vi "PXI-Compute DI Skip Samples.vi"(0 "AO Tasks":T1[](array[typedef]), 7 "DI Tasks":T1[](array[typedef]), 11 "error in (no error)":errorcluster) -> (4 "Skip Samples":i32, 15 "error out":errorcluster)   [LabVIEW 2020]
doc: "Determines the number of AI samples to skip in order to register AO and AI (accounting for the latencies of the 24-bit boards)."
uses:
  Type Defs/Task Struct.ctl
  PXI Globals.vi
panel:
  out "Any 16-bit AI?":bool
  out "Any 16-bit AO?":bool
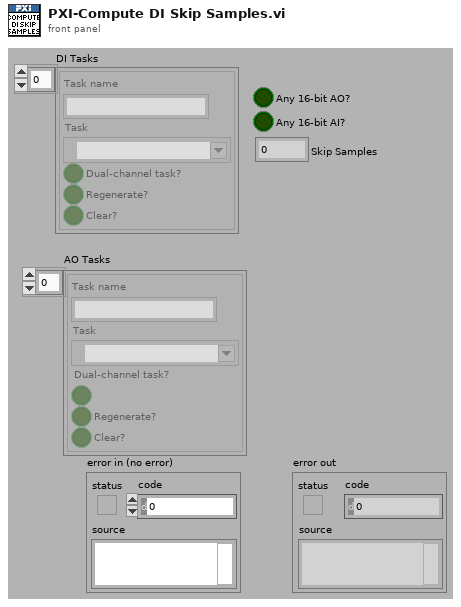
[diagram p1: front panel]
types:
  T1 = typedef "Task Struct.ctl" = cluster{"Task name":string, "Task":refnum<k21>, "Dual-channel task?":bool, "Regenerate?":bool, "Clear?":bool}
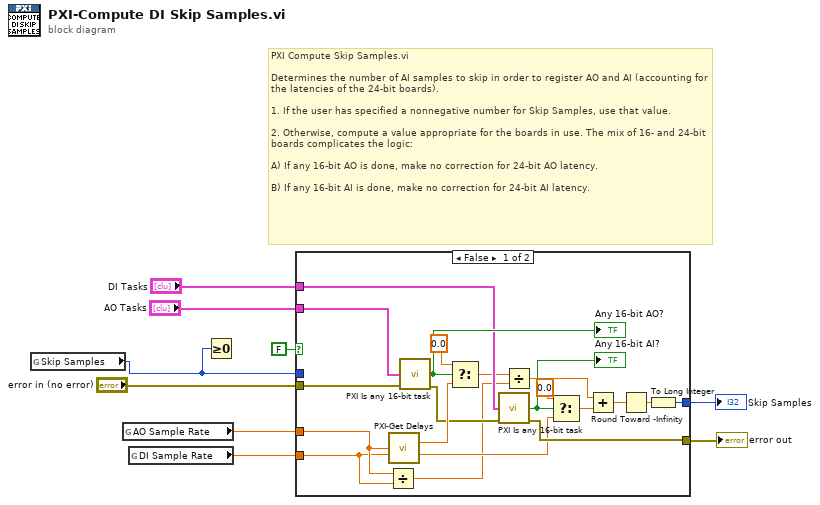
[diagram p0: block diagram]
diagram:
  # "PXI Compute Skip Samples.vi\n\nDetermines the number of AI samples to skip in order to register AO and AI (accounting for the latencies of the 24-bit boards). \n\n1. If the user has specified a nonnegative number for Skip Samples, use that value. \n\n2. Otherwise, compute a value appropriate for the boards in use. The mix of 16- and 24-bit boards complicates the logic:\n\nA) If any 16-bit AO is done, make no correction for 24-bit AO latency.\n\nB) If any 16-bit AI is done, make no correction for 24-bit AI latency."
  n1 = global read "PXI Globals.vi" "Skip Samples"() -> (w7:i32)
  n2 = global read "PXI Globals.vi" "AO Sample Rate"() -> (w5:dbl)
  n3 = global read "PXI Globals.vi" "DI Sample Rate"() -> (w4:dbl)
  n4 = Greater Or Equal To 0?(x=w7) -> ()  [unwired: 1 out]
  n5 = case shown="False" FALSE {
    tunnel: "error in (no error)" -> [w10 w31]
    tunnel: [w27 w30] -> w3
    tunnel: [w20 w31] -> w9
    tunnel: w7 -> [_ w30]
    tunnel: "AO Tasks" -> [w26 _]
    tunnel: "DI Tasks" -> [w21 _]
    tunnel: w5 -> [w12 _]
    tunnel: w4 -> [w11 _]
    frame False {
      n6 = Divide(x=w12, y=w11) -> (x/y=w13:dbl)
      n7 = call "PXI-Get Delays.vi"("AO Rate (Samples/s)"=w12, "AI Rate (Samples/s)"=w11) -> ("AO delay (samples)"=w23:dbl, "AI delay (samples)"=w18:dbl)  [unwired: 12 in]
      n8 = call "PXI Is any 16-bit task.vi"("Task Array"=w26, "error in (no error)"=w10) -> ("Any 16-bit task?"=w25:bool, "error out"=w22:errorcluster)  [unwired: 12 in]
      "Any 16-bit AO?" <- w25
      n9 = Select(t=0.0 ("f"), s=w25, f=w23) -> (s? t:f=w15:dbl)
      n10 = call "PXI Is any 16-bit task.vi"("Task Array"=w21, "error in (no error)"=w22) -> ("Any 16-bit task?"=w19:bool, "error out"=w20:errorcluster)  [unwired: 12 in]
      "Any 16-bit AI?" <- w19
      n11 = Divide(x=w15, y=w13) -> (x/y=w14:dbl)
      n12 = Select(t=0.0, s=w19, f=w18) -> (s? t:f=w16:dbl)
      n13 = Add(x=w14, y=w16) -> (x+y=w28:dbl)
      n14 = Round Toward -Infinity(1:w28) -> (0:w29:dbl)
      n15 = To Long Integer(number=w29) -> (32bit integer=w27:i32)
    }
    frame True {
    }
  }
  "error out" <- w9
  "Skip Samples" <- w3
